vi "Menu -- About Display.vi"(8 "error in":errorcluster) -> (0 "error out":errorcluster)   [LabVIEW 2016, in "CML UI.lvlib"]
doc: "<b>Note:</b> This VI was modified by the <b>Validate DQMH Module</b> tool to turn off automatic error handling."
uses:
  CML UI.lvlib
panel:
  out "String input":string="The Application"
  in  "OK Button":bool
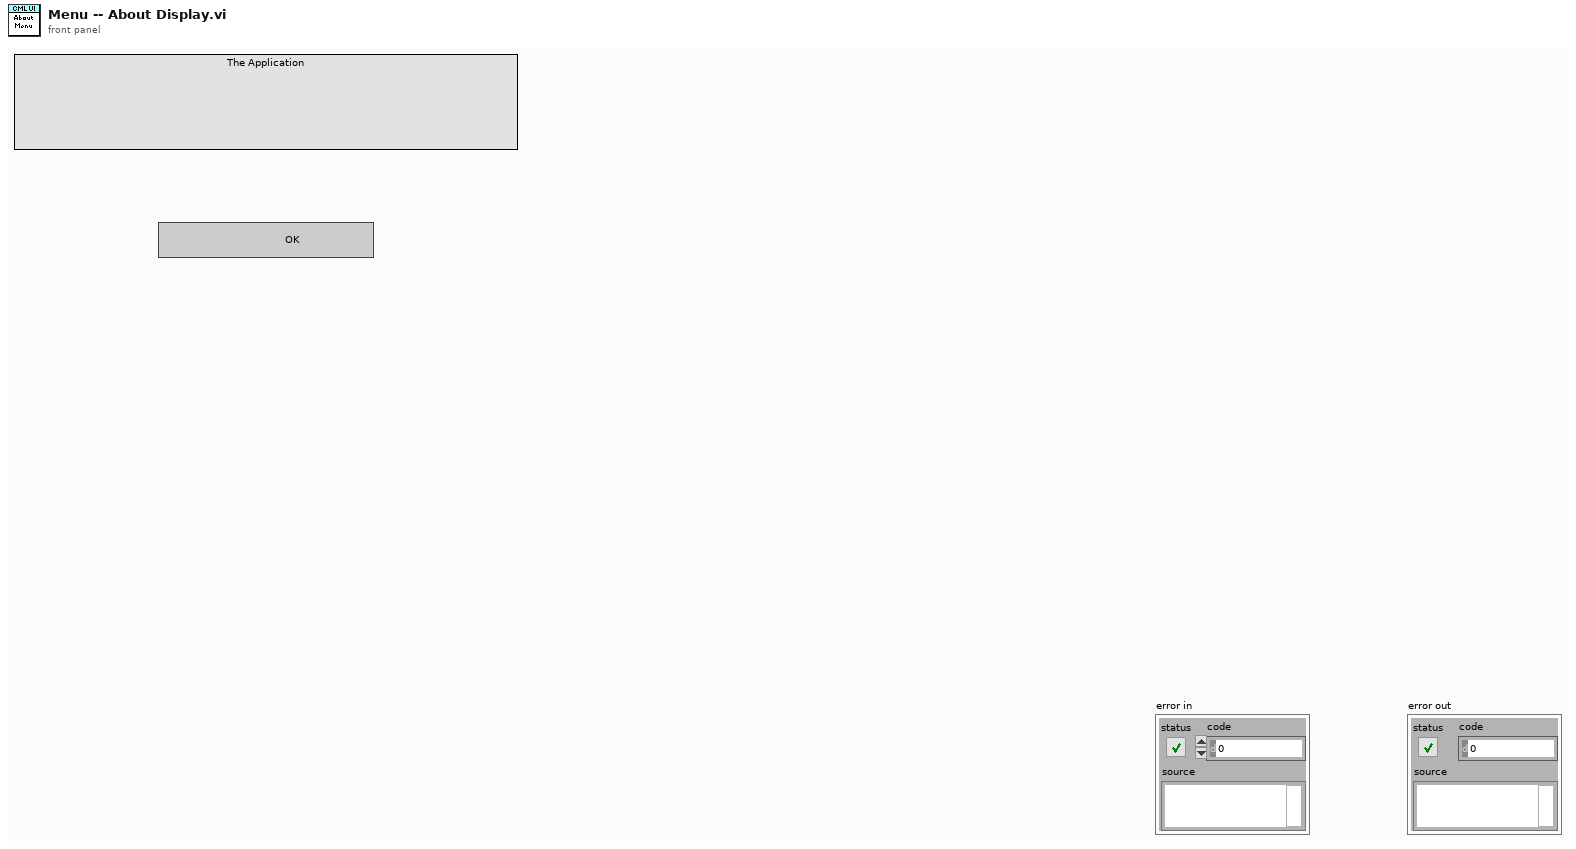
[diagram p1: front panel]
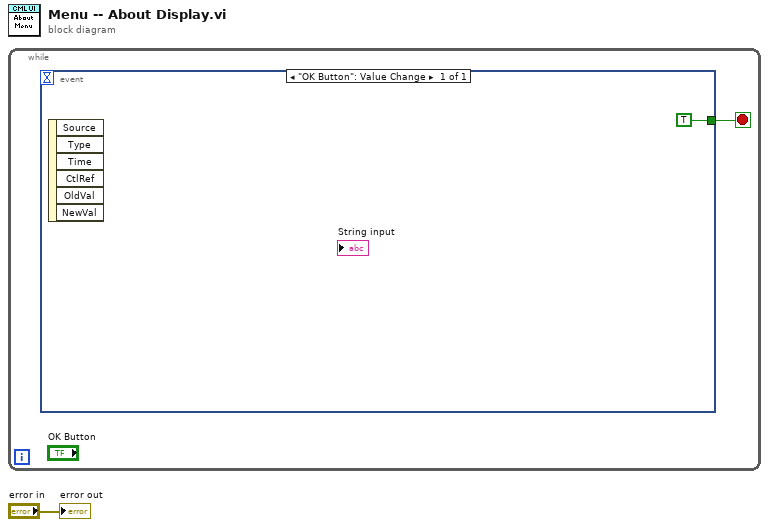
[diagram p0: block diagram]
diagram:
  n1 = while {
    stop <- w2 stop-if-true
    n2 = event shown="[0] \"OK Button\": Value Change" {
      selector: _ -> [_]
      dyn-events: _ -> [_]
      timeout: _ -> [_]
      tunnel: [TRUE] -> w2
      event "OK Button": Value Change {
        n3 = event-data() -> ()  [unwired: 1 in, 6 out]
      }
    }
  }
  "error out" <- "error in"
